vi "IMMU - Initialise Magnetometer.vi"(8 "error in (no error)":errorcluster) -> ()   [LabVIEW 2021]
uses:
  <vilib>/myRIO/Instrument Drivers/Onboard IO/I2C/typedefs/I2C User Configuration.ctl
  <vilib>/myRIO/Instrument Drivers/Onboard IO/I2C/typedefs/I2C Transfer Rate.ctl
  <vilib>/myRIO/Instrument Drivers/Onboard IO/I2C/typedefs/I2C Reference.ctl
  <vilib>/myRIO/Common/Instrument Driver Framework/Utilities/typedefs/myRIO Generic Hardware Reference.ctl
  <vilib>/myRIO/Common/Instrument Driver Framework/Utilities/typedefs/Hardware Version Enum.ctl
  <vilib>/myRIO/Common/Instrument Driver Framework/Utilities/typedefs/myRIO v1.0 Reference.ctl
  <vilib>/myRIO/Common/Instrument Driver Framework/Utilities/typedefs/Generic FPGA Reference.ctl
  <vilib>/myRIO/Common/Instrument Driver Framework/myRIO v1.0/I2C/typedefs/I2C Channels Enum.ctl
  <vilib>/myRIO/Instrument Drivers/Onboard IO/I2C/typedefs/I2C Configuration.ctl
  <vilib>/userDefined/High Color/nirio_resource_hc.ctl
  <vilib>/myRIO/Common/Instrument Driver Framework/Utilities/vis/Is FPGA Ref Available.vi
  <vilib>/myRIO/Common/Instrument Driver Framework/myRIO v1.0/I2C/vis/myRIO v1.1 Open I2C.vi
  <vilib>/myRIO/Instrument Drivers/Onboard IO/I2C/vis/Configure.vi
  <vilib>/myRIO/Instrument Drivers/Onboard IO/I2C/vis/Write.vi
  <vilib>/myRIO/Instrument Drivers/Onboard IO/I2C/vis/Write Read.vi
  <vilib>/myRIO/Common/Instrument Driver Framework/Utilities/vis/Validate Channels.vi
  <vilib>/myRIO/Common/Instrument Driver Framework/myRIO v1.0/I2C/vis/myRIO v1.0 Reserve I2C.vi
  <vilib>/myRIO/Common/Instrument Driver Framework/myRIO v1.0/I2C/vis/myRIO v1.0 Build MUX Configuration I2C.vi
  <vilib>/myRIO/Common/Instrument Driver Framework/myRIO v1.0/Resource Manager/vis/myRIO v1.0 Reserve Channel List.vi
  <vilib>/myRIO/Common/Instrument Driver Framework/myRIO v1.0/Resource Manager/vis/myRIO v1.0 Create Configuration List.vi
  <vilib>/myRIO/Common/Instrument Driver Framework/myRIO v1.0/Resource Manager/vis/myRIO v1.0 Reserve Channel.vi
  <vilib>/myRIO/Common/Instrument Driver Framework/myRIO v1.0/Resource Manager/vis/myRIO v1.0 Unreserve Channel.vi
  <vilib>/myRIO/Common/Instrument Driver Framework/myRIO v1.0/Resource Manager/vis/myRIO v1.0 Build Mutex Name.vi
  <vilib>/Utility/VariantDataType/GetNumericInfo.vi
  <vilib>/Utility/error.llb/Error Cluster From Error Code.vi
  <vilib>/myRIO/Common/Instrument Driver Framework/myRIO v1.0/myRIO v1.1 Open.vi
  <vilib>/myRIO/Common/Instrument Driver Framework/Utilities/vis/IO Manager.vi
  <vilib>/myRIO/Common/Instrument Driver Framework/Utilities/vis/Configuration Manager.vi
  <vilib>/myRIO/Common/Instrument Driver Framework/myRIO v1.0/Resource Manager/vis/myRIO v1.0 Configure IO.vi
  <vilib>/myRIO/Common/Instrument Driver Framework/myRIO v1.0/myRIO v1.0 Close.vi
  <vilib>/myRIO/Common/Instrument Driver Framework/myRIO v1.0/I2C/vis/myRIO v1.0 Configure I2C.vi
  <vilib>/myRIO/Common/Instrument Driver Framework/myRIO v1.0/I2C/vis/myRIO v1.0 Write I2C.vi
  <vilib>/myRIO/Common/Instrument Driver Framework/myRIO v1.0/I2C/vis/myRIO v1.0 Read I2C.vi
  <vilib>/myRIO/Express VI/Onboard IO/I2C/I2C Express VI.xnode
  <vilib>/myRIO/Instrument Drivers/Onboard IO/I2C/vis/myRIO I2C Open.xnode
  <vilib>/myRIO/Instrument Drivers/Onboard IO/I2C/I2C.lvlib
panel:
  out "Ext Data Out":u8[](array[numeric])
  out "Who am I":u8[](array[numeric])
  out "Bytes Read":u8[](array[numeric])
  out "Bytes Read 2":u8[](array[numeric])
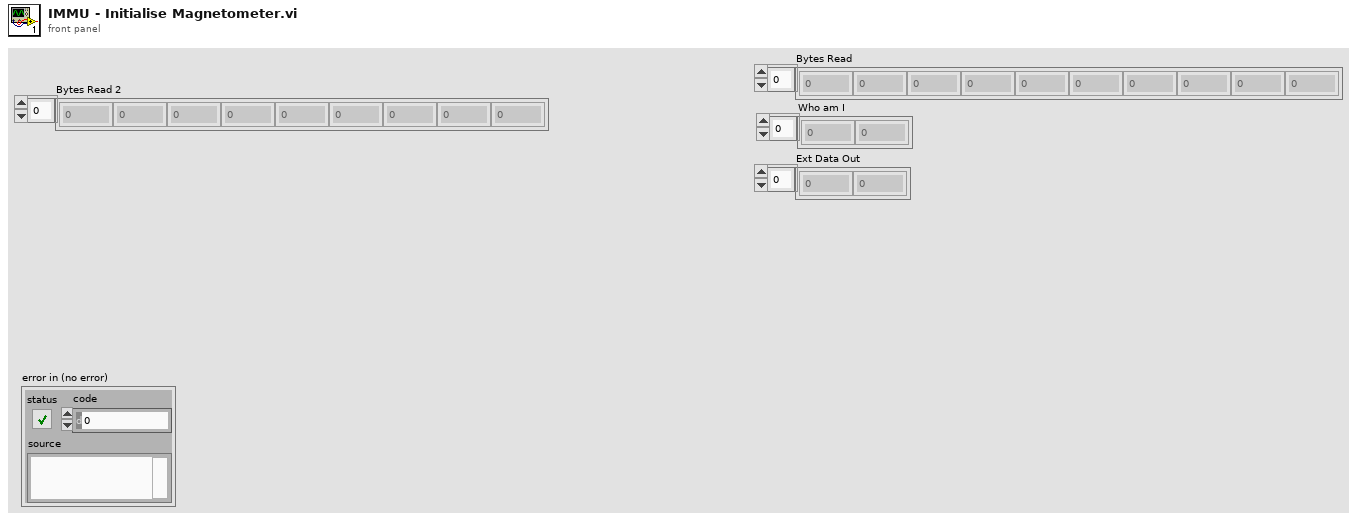
[diagram p1: front panel]
types:
  T1 = typedef "I2C.lvlib/I2C Reference.ctl" = cluster{"myRIO Reference":T2, "I2C Channels Enum":T6, "I2C Configuration":T7}
  T2 = typedef "myRIO Generic Hardware Reference.ctl" = cluster{"myRIO Model":T3, "myRIO Hardware Reference":T4}
  T3 = typedef "Hardware Version Enum.ctl" = enum16{"Unknown", "myRIO-1900", "myRIO-1950", "roboRIO", "NI ELVIS RIO CM", "ELVIS III"}
  T4 = typedef "myRIO v1.0 Reference.ctl" = cluster{"Generic FPGA Reference":T5, "Allow multiple opens":bool}
  T5 = typedef "Generic FPGA Reference.ctl" = refnum<k20>
  T6 = typedef "I2C Channels Enum.ctl" = enum16{"Not Connected", "A/I2C", "B/I2C", "I2C/I2C"}
  T7 = typedef "I2C.lvlib/I2C Configuration.ctl" = cluster{"I2C Transfer Rate":T8}
  T8 = typedef "I2C.lvlib/I2C Transfer Rate.ctl" = enum16{"Standard mode (100 kbps)", "Fast mode (400 kbps)"}
  T9 = typedef "I2C.lvlib/I2C User Configuration.ctl" = cluster{"I2C Transfer Rate":T8}
  T10 = typedef "nirio_resource_hc.ctl" = tag
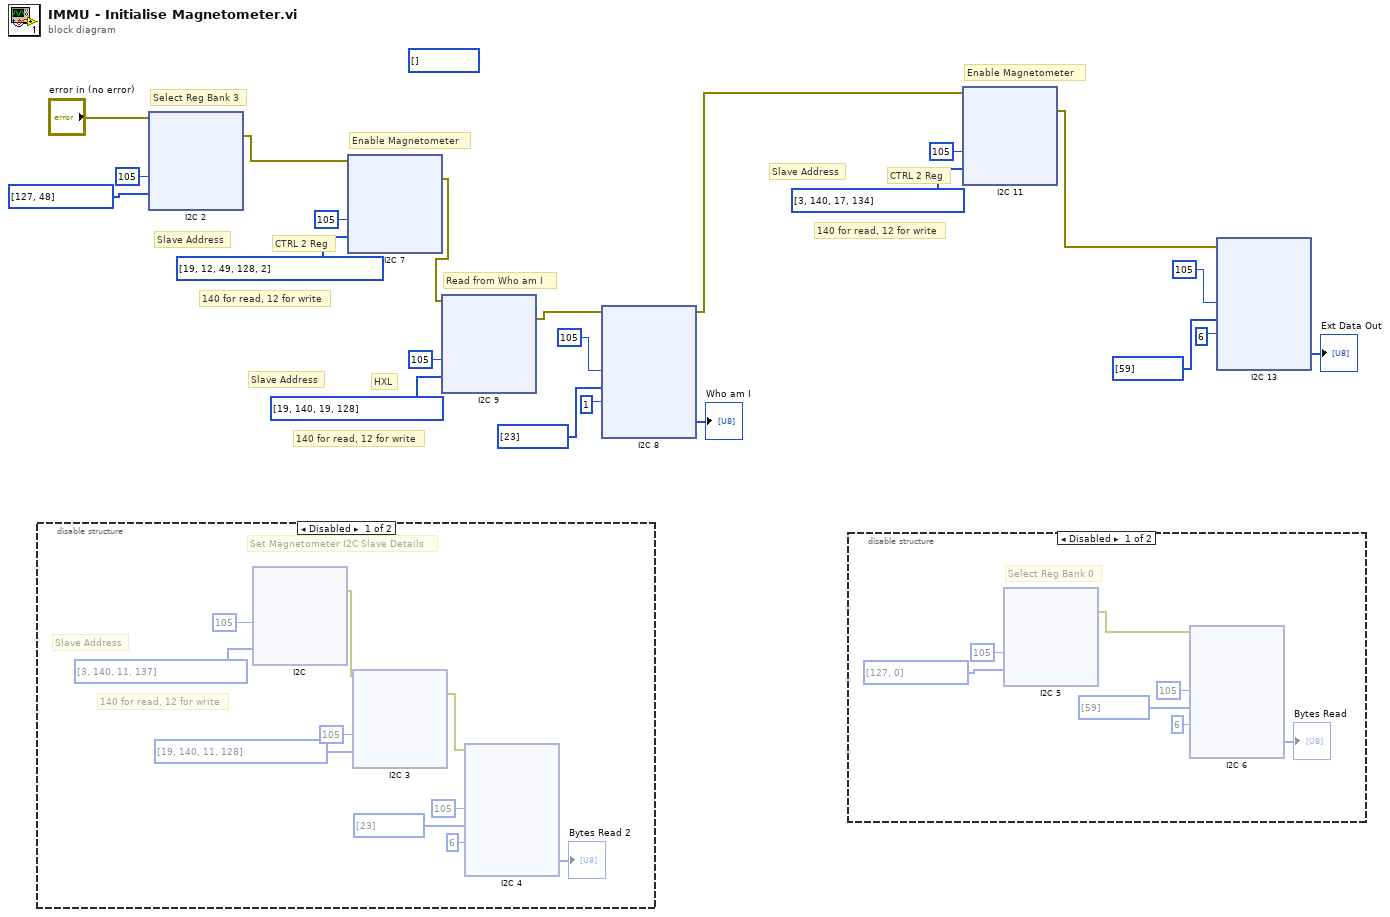
[diagram p0: block diagram]
diagram:
  (unwired) u8[] []
  # "CTRL 2 Reg"
  # "Slave Address"
  # "140 for read, 12 for write"
  # "Enable Magnetometer"
  # "HXL"
  # "CTRL 2 Reg"
  # "Slave Address"
  # "140 for read, 12 for write"
  # "Read from Who am I"
  # "Slave Address"
  # "140 for read, 12 for write"
  # "Enable Magnetometer"
  # "Select Reg Bank 3"
  n1 = disable-structure shown="Disabled" {
    frame Disabled {
      # "Slave Address"
      # "140 for read, 12 for write"
      # "Set Magnetometer I2C Slave Details"
      n2 = xnode "I2C"("Slave Address (7-bit)"=u8 105, "Bytes to Write"=u8[] [3, 140, 11, 137]) -> ("error out"=w24:errorcluster)  [unwired: 1 in]
      n3 = xnode "I2C 3"("Slave Address (7-bit)"=u8 105, "Bytes to Write"=u8[] [19, 140, 11, 128], "error in (no error)"=w24) -> ("error out"=w23:errorcluster)
      n4 = xnode "I2C 4"("Slave Address (7-bit)"=u8 105, "Bytes to Write"=u8[] [23], "Byte Count"=u32 6, "error in (no error)"=w23) -> ("Bytes Read"=→"Bytes Read 2":u8[])  [unwired: 1 out]
    }
    frame Enabled {
    }
  }
  n5 = xnode "I2C 2"("Slave Address (7-bit)"=u8 105, "Bytes to Write"=u8[] [127, 48], "error in (no error)"="error in (no error)") -> ("error out"=w9:errorcluster)
  n6 = xnode "I2C 7"("Slave Address (7-bit)"=u8 105, "Bytes to Write"=u8[] [19, 12, 49, 128, 2], "error in (no error)"=w9) -> ("error out"=w11:errorcluster)
  n7 = xnode "I2C 9"("Slave Address (7-bit)"=u8 105, "Bytes to Write"=u8[] [19, 140, 19, 128], "error in (no error)"=w11) -> ("error out"=w12:errorcluster)
  n8 = xnode "I2C 8"("Slave Address (7-bit)"=u8 105, "Bytes to Write"=u8[] [23], "Byte Count"=u32 1, "error in (no error)"=w12) -> ("Bytes Read"=→"Who am I":u8[], "error out"=w2:errorcluster)
  n9 = disable-structure shown="Disabled" {
    frame Disabled {
      # "Select Reg Bank 0"
      n10 = xnode "I2C 5"("Slave Address (7-bit)"=u8 105, "Bytes to Write"=u8[] [127, 0]) -> ("error out"=w150:errorcluster)  [unwired: 1 in]
      n11 = xnode "I2C 6"("Slave Address (7-bit)"=u8 105, "Bytes to Write"=u8[] [59], "Byte Count"=u32 6, "error in (no error)"=w150) -> ("Bytes Read"=→"Bytes Read":u8[])  [unwired: 1 out]
    }
    frame Enabled {
    }
  }
  n12 = xnode "I2C 11"("Slave Address (7-bit)"=u8 105, "Bytes to Write"=u8[] [3, 140, 17, 134], "error in (no error)"=w2) -> ("error out"=w1:errorcluster)
  n13 = xnode "I2C 13"("Slave Address (7-bit)"=u8 105, "Bytes to Write"=u8[] [59], "Byte Count"=u32 6, "error in (no error)"=w1) -> ("Bytes Read"=→"Ext Data Out":u8[])  [unwired: 1 out]
